vi "playing with images 1.vi"() -> ()   [LabVIEW 2018]
panel:
  in  "Numeric":dbl
  in  "Numeric 2":dbl
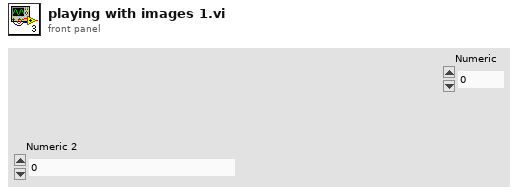
[diagram p1: front panel]
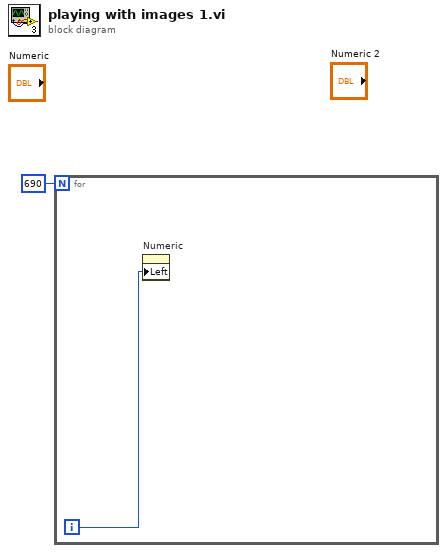
[diagram p0: block diagram]
diagram:
  n1 = for {
    N: 690 -> [_]
    i -> [w2]
    n2 = property on="Numeric" class="DigNum (strict)"("Left"=w2) -> ()  [unwired: 2 in, 2 out]
  }
